vi "subUpdateInstallPath.vi"(8 "error in (no error)":errorcluster, 10 "New VS InstallPath":string, 11 "DOM document in":refnum<k20>) -> (0 "error out":errorcluster, 3 "DOM document out":refnum<k20>)   [LabVIEW 2015, in "veristand-steps-build-tools.lvlib"]
uses:
  <userlib>/Simple XML/_polymorphics/Create Tag - Child with Text.vi
  <vilib>/xml/Close Reference(Node).vi
  veristand-steps-build-tools.lvlib
  <vilib>/xml/NI_XML.lvlib
  <resource>/objmgr/DOMUserDefRef.rc
  <userlib>/Simple XML/Simple XML.lvlib
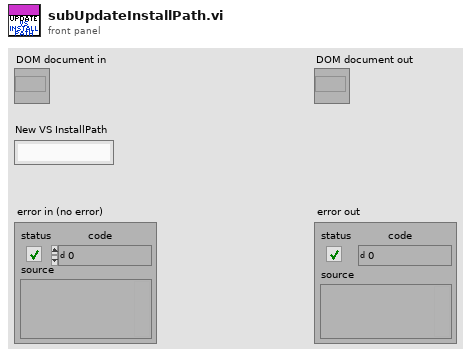
[diagram p1: front panel]
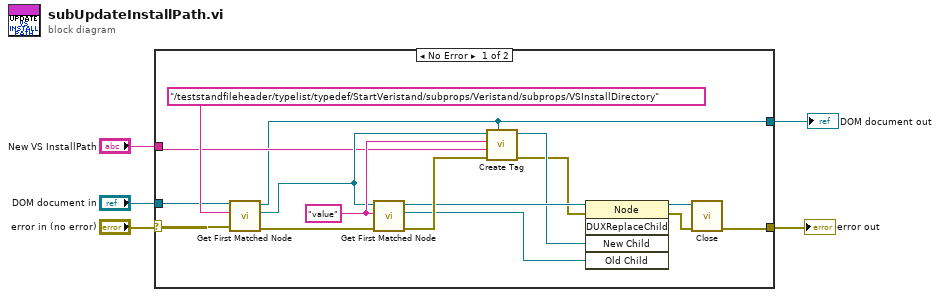
[diagram p0: block diagram]
diagram:
  n1 = case shown="No Error" "error in (no error)" {
    selector: "error in (no error)" -> [w21 w23]
    tunnel: [w10 w23] -> w4
    tunnel: "DOM document in" -> [w19 w22]
    tunnel: [w6 w22] -> w2
    tunnel: "New VS InstallPath" -> [w7 _]
    frame No Error {
      w13 = "value" ("XPath expression")
      n2 = call <vilib>:"Get First Matched Node.vi"("error in (no error)"=w21, "XPath expression"="/teststandfileheader/typelist/typedef/StartVeristand/subprops/Veristand/subprops/VSInstallDirectory", "node in"=w19) -> ("error out"=w8:errorcluster, "node result"=w9:refnum<k20>, "node out"=w6:refnum<k20>)  [unwired: 6 in]
      n3 = call <vilib>:"Get First Matched Node.vi"("error in (no error)"=w8, "XPath expression"=w13, "node in"=w9) -> ("error out"=w16:errorcluster, "node result"=w11:refnum<k20>, "node out"=w15:refnum<k20>)  [unwired: 6 in]
      n4 = call-poly <userlib>:"Create Tag.vi"("DOM document reference"=w6, "error in (no error)"=w16, "Text Data"=w7, "Tag Name"=w13, "Parent Element reference"=w9) -> ("error out"=w12:errorcluster, "Child Element reference"=w14:refnum<k20>)  [unwired: 5 in]
      n5 = invoke class="Node" method="DUXReplaceChild"(reference=w15, error in=w12, "New Child"=w14, "Old Child"=w11) -> (reference out=w18:refnum<k20>, error out=w17:errorcluster)  [unwired: 1 in, 3 out]
      n6 = call-poly <vilib>:"Close.vi"("error in (no error)"=w17, "node"=w18) -> ("error out"=w10:errorcluster)  [unwired: 7 in]
    }
    frame Error {
    }
  }
  "DOM document out" <- w2
  "error out" <- w4
